vi "Seq Dialog Read File.vi"(8 "Segment Data":T1) -> (0 "Step Hisitory":string[](array[string]), 3 "Segment Data 2":T1, 4 "Add Step?":bool)   [LabVIEW 2018]
uses:
  type defs/Sequence Info.ctl
panel:
  in  "Select Flash File":path
  out "String 2":string="Pre Run Station - Glass - Vent Open"
  in  "Description":string
  in  "Save":bool
  in  "Cancel":bool
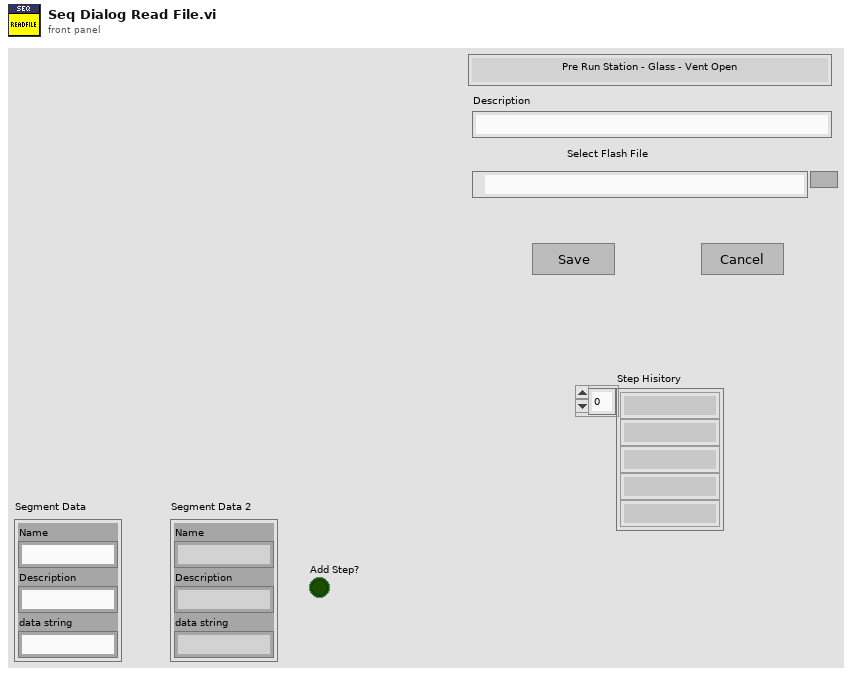
[diagram p1: front panel]
types:
  T1 = typedef "Sequence Info.ctl" = cluster{"Name":string, "Description":string, "data string":string}
  T2 = cluster{"Segment Data":T1, "Add Step?":bool, "Old Data":string, "New Data":string}
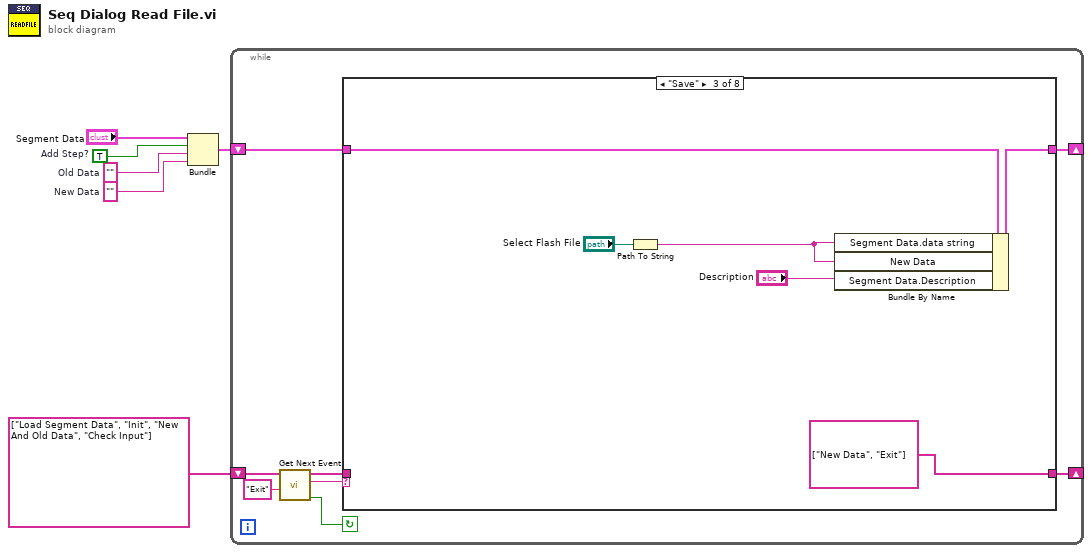
[diagram p0: block diagram]
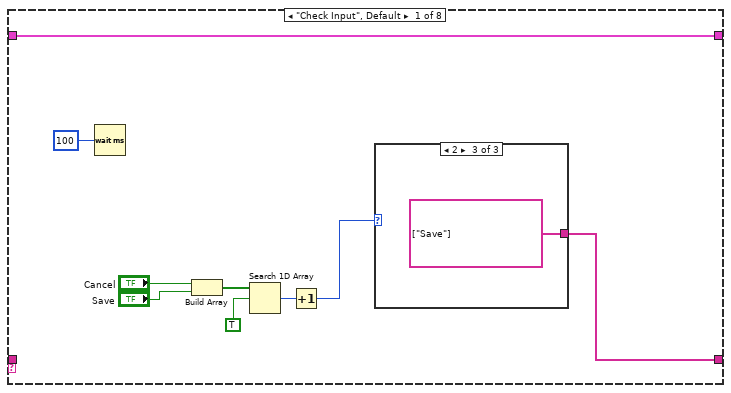
[diagram p2: hidden frame]
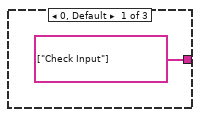
[diagram p3: hidden frame]
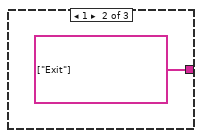
[diagram p4: hidden frame]
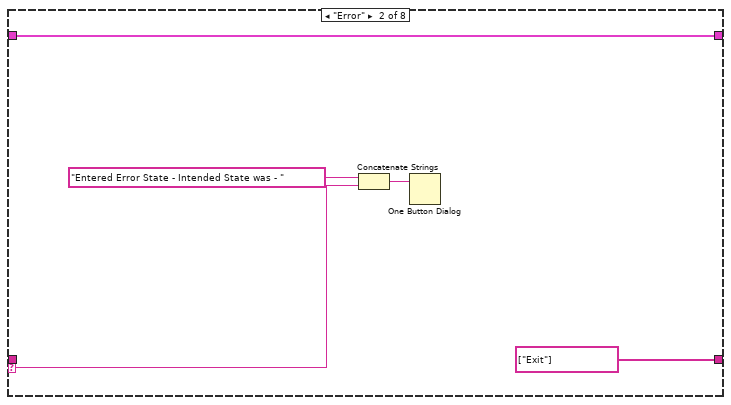
[diagram p5: hidden frame]
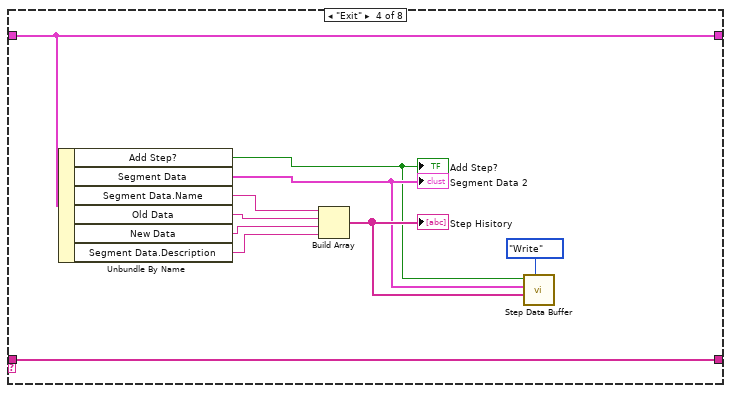
[diagram p6: hidden frame]
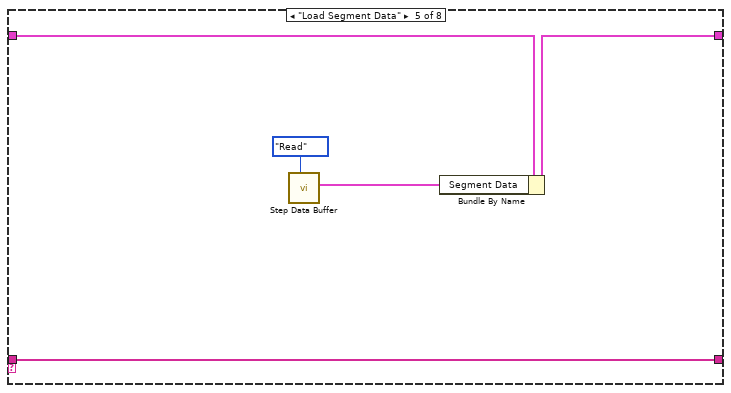
[diagram p7: hidden frame]
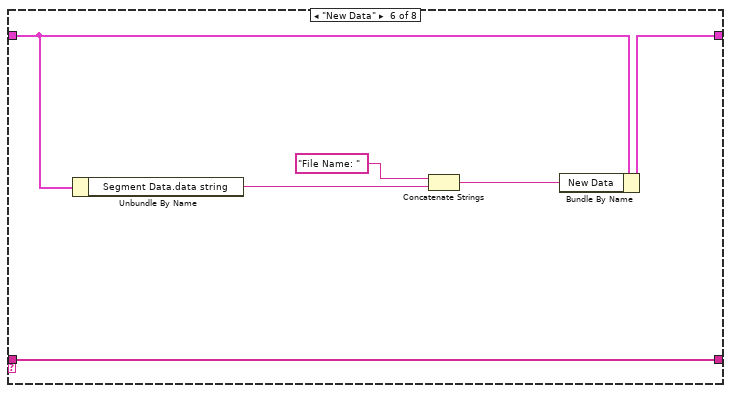
[diagram p8: hidden frame]
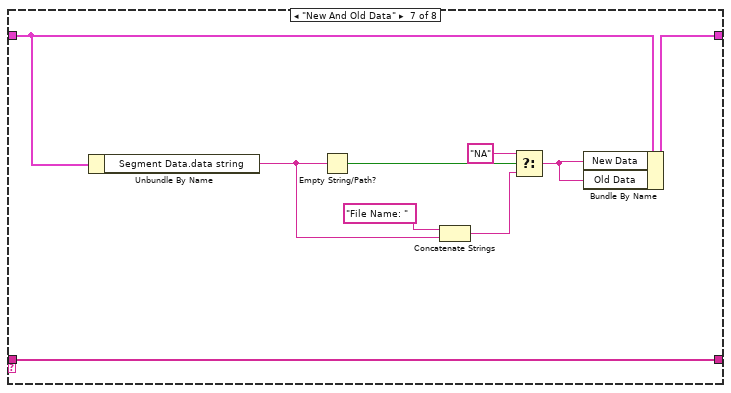
[diagram p9: hidden frame]
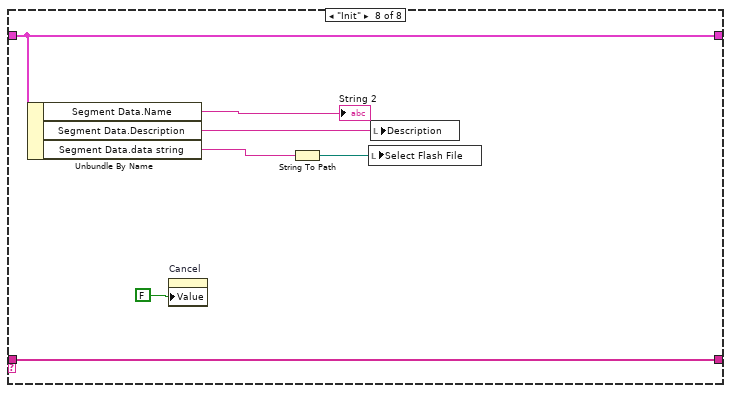
[diagram p10: hidden frame]
diagram:
  w2 = ""  # New Data
  w3 = ""  # Old Data
  w4 = TRUE  # Add Step?
  n1 = Bundle("Segment Data"="Segment Data", "Add Step?"=w4, "Old Data"=w3, "New Data"=w2) -> (w5:T2)  [unwired: 1 in]
  n2 = while {
    shift-right: [w12] -> _
    shift-left: string[] ["Load Segment Data", "Init", "New And Old Data", "Check Input"] ("Event queue out") -> [w11]
    shift-right: [w7] -> _
    shift-left: w5 -> [w8]
    stop <- w10 continue-if-true
    n3 = call "Get Next Event.vi"("Exit Event"="Exit", "event queue in"=w11) -> ("Condition (Exit:F)"=w10:bool, "next event"=w14:string, "event queue out"=w13:string[])  [unwired: 3 in]
    n4 = case shown="\"Save\"" w14 {
      selector: w14 -> [_ w28 _ _ _ _ _ _]
      tunnel: w13 -> [_ _ _ w47 w52 w56 w66 w74]
      tunnel: [w17 string[] ["Exit"] ("event queue out") string[] ["New Data", "Exit"] ("Event queue out") w47 w52 w56 w66 w74] -> w12
      tunnel: w8 -> [w22 w31 w35 w43 w49 w55 w61 w72]
      tunnel: [w22 w31 w37 w43 w48 w54 w60 w72] -> w7
      frame "Check Input", Default {
        n5 = Wait (ms)(milliseconds to wait=u32 100) -> ()  [unwired: 1 out]
        n6 = Build Array("Cancel", "Save") -> (w19:bool[])
        n7 = Search 1D Array(1D array=w19, element=TRUE) -> (index of element=w20:i32)  [unwired: 1 in]
        n8 = Increment(x=w20) -> (x+1=w21:i32)
        n9 = case shown="2" w21 {
          tunnel: [string[] ["Check Input"] ("Events to Insert") string[] ["Exit"] ("Events to Insert") string[] ["Save"] ("Events to Insert")] -> w17
          frame 0, Default {
          }
          frame 1 {
          }
          frame 2 {
          }
        }
      }
      frame "Error" {
        n10 = Concatenate Strings("Entered Error State - Intended State was - " ("string"), w28) -> (w30:string)
        n11 = One Button Dialog(message=w30) -> ()  [unwired: 1 in, 1 out]
      }
      frame "Save" {
        n12 = Path To String(path="Select Flash File") -> (string=w32:string)
        n13 = Bundle By Name(cluster=w35, "Segment Data.data string"=w32, "New Data"=w32, "Segment Data.Description"="Description") -> (w37:T2)
      }
      frame "Exit" {
        n14 = Unbundle By Name(w43) -> ("Add Step?"=w39:bool, "Segment Data"=w40:T1, "Segment Data.Name"=w45:string, "Old Data"=w44:string, "New Data"=w46:string, "Segment Data.Description"=w38:string)
        "Segment Data 2" <- w40
        "Add Step?" <- w39
        n15 = Build Array(w45, w44, w46, w38) -> (w41:string[])
        "Step Hisitory" <- w41
        n16 = call "Step Data Buffer.vi"("Mode"=enum16{"Init", "Read", "Write"}."Write", "Step Hisitory In"=w41, "Segment Data In"=w40, "Add Step? In"=w39) -> ()  [unwired: 3 in, 5 out]
      }
      frame "Load Segment Data" {
        n17 = call "Step Data Buffer.vi"("Mode"=enum16{"Init", "Read", "Write"}."Read") -> ("Segment Data Out"=w51:T1)  [unwired: 6 in, 4 out]
        n18 = Bundle By Name(cluster=w49, "Segment Data"=w51) -> (w48:T2)
      }
      frame "New Data" {
        n19 = Unbundle By Name(w55) -> ("Segment Data.data string"=w53:string)
        n20 = Concatenate Strings("File Name: " ("string"), w53) -> (w57:string)
        n21 = Bundle By Name(cluster=w55, "New Data"=w57) -> (w54:T2)
      }
      frame "New And Old Data" {
        n22 = Unbundle By Name(w61) -> ("Segment Data.data string"=w59:string)
        n23 = Empty String/Path?(string/path=w59) -> (empty?=w65:bool)
        n24 = Concatenate Strings("File Name: " ("string"), w59) -> (w62:string)
        n25 = Select(t="NA", s=w65, f=w62) -> (s? t:f=w63:string)
        n26 = Bundle By Name(cluster=w61, "New Data"=w63, "Old Data"=w63) -> (w60:T2)
      }
      frame "Init" {
        n27 = Unbundle By Name(w72) -> ("Segment Data.Name"=→"String 2":string, "Segment Data.Description"=w73:string, "Segment Data.data string"=w71:string)
        n28 = property on="Cancel" class="Bool (严格)"("Value"=FALSE ("Cancel")) -> ()  [unwired: 2 in, 2 out]
        n29 = String To Path(string=w71) -> (path=w70:path)
        n30 = local write "Select Flash File"(w70) -> ()
        n31 = local write "Description"(w73) -> ()
      }
    }
  }
